vi "ClickOnSquereOperations.vi"(9 "Input DataBase":T1, 10 "Off Board?":bool, 11 "Clicked Position":i32[](array[numeric])) -> (2 "Output DataBase":T1, 3 "Output State":T8)   [LabVIEW 2019]
uses:
  #typedef_DataBase.ctl
  #typedef_SquareType.ctl
  #typedef_Color.ctl
  #typedef_Piece.ctl
  #typedef_PieceType.ctl
  #typedef_SquareLook.ctl
  #typedef_SpecialMoves.ctl
  #typedef_ProgramStates.ctl
panel:
  out "?":u16[][](array[ring])
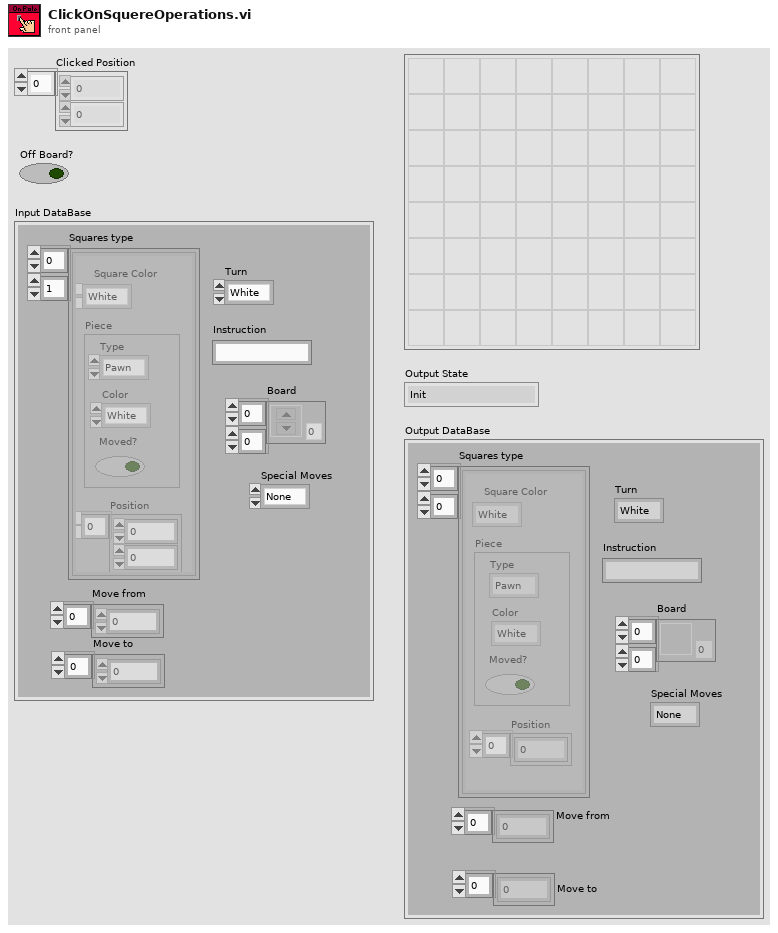
[diagram p1: front panel]
types:
  T1 = typedef "#typedef_DataBase.ctl" = cluster{"Squares type":T2[][], "Turn":T3, "Move from":i32[], "Move to":i32[], "Instruction":string, "Board":T6[][], "Special Moves":T7}
  T2 = typedef "#typedef_SquareType.ctl" = cluster{"Square Color":T3, "Position":i32[], "Piece":T4}
  T3 = typedef "#typedef_Color.ctl" = enum16{"White", "Black"}
  T4 = typedef "#typedef_Piece.ctl" = cluster{"Type":T5, "Color":T3, "Moved?":bool}
  T5 = typedef "#typedef_PieceType.ctl" = enum16{"None", "Pawn", "Knight", "Bishop", "Rook", "Queen", "King"}
  T6 = typedef "#typedef_SquareLook.ctl" = u16
  T7 = typedef "#typedef_SpecialMoves.ctl" = enum16{"None", "Last Square", "Beat in the Passage", "Short Castle", "Long Castle"}
  T8 = typedef "#typedef_ProgramStates.ctl" = enum16{"Init", "Clicking on Piece", "Clicking on Square", "Checking Movement", "Checking King  ", "Checking if Mate", "End"}
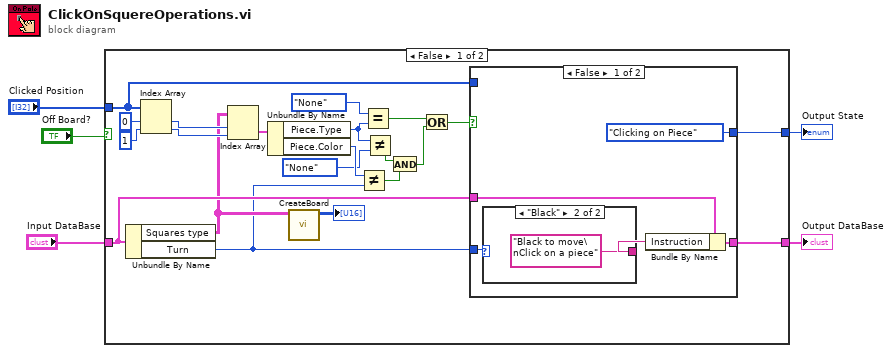
[diagram p0: block diagram]
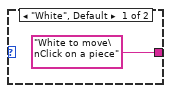
[diagram p2: hidden frame]
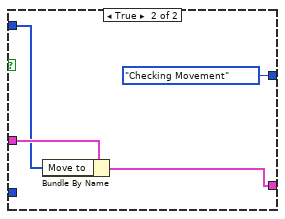
[diagram p3: hidden frame]
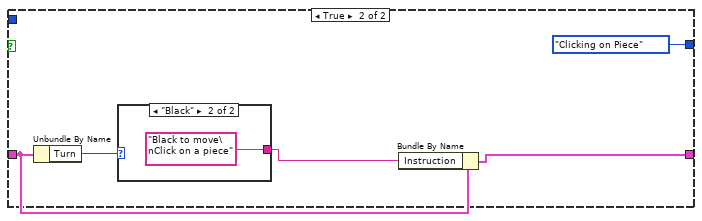
[diagram p4: hidden frame]
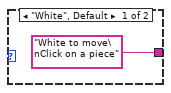
[diagram p5: hidden frame]
diagram:
  n1 = case shown="False" "Off Board?" {
    tunnel: "Input DataBase" -> [w19 w40]
    tunnel: [w18 w38] -> w1
    tunnel: [w20 #typedef_ProgramStates."Clicking on Piece" ("Conditional State")] -> w2
    tunnel: "Clicked Position" -> [w15 _]
    frame False {
      n2 = Unbundle By Name(w19) -> ("Squares type"=w17:T2[][], "Turn"=w12:T3)
      n3 = Index Array(array=w15, index #1=0 ("index"), index #2=1 ("index")) -> (element #1=w24:i32, element #2=w23:i32)
      n4 = Index Array(array=w17, index (row)=w24, index (col)=w23) -> (element=w22:T2)
      n5 = Unbundle By Name(w22) -> ("Piece.Type"=w14:T5, "Piece.Color"=w13:T3)
      n6 = call "CreateBoard.vi"("Squares type"=w17) -> ("Board"=→"?":u16[][])  [unwired: 10 in]
      n7 = Not Equal?(x=w13, y=w12) -> (x != y?=w10:bool)
      n8 = Equal?(x=#typedef_PieceType."None", y=w14) -> (x = y?=w6:bool)
      n9 = Not Equal?(x=w14, y=#typedef_PieceType."None") -> (x != y?=w9:bool)
      n10 = And(x=w9, y=w10) -> (x .and. y?=w7:bool)
      n11 = Or(x=w6, y=w7) -> (x .or. y?=w8:bool)
      n12 = case shown="False" w8 {
        tunnel: [#typedef_ProgramStates."Clicking on Piece" ("Conditional State") #typedef_ProgramStates."Checking Movement" ("Conditional State")] -> w20
        tunnel: w19 -> [w30 w37]
        tunnel: [w29 w36] -> w18
        tunnel: w15 -> [_ w34]
        tunnel: w12 -> [w28 _]
        frame False {
          n13 = case shown="\"Black\"" w28 {
            tunnel: ["White to move\nClick on a piece" "Black to move\nClick on a piece"] -> w27
            frame "White", Default {
            }
            frame "Black" {
            }
          }
          n14 = Bundle By Name(cluster=w30, "Instruction"=w27) -> (w29:T1)
        }
        frame True {
          n15 = Bundle By Name(cluster=w37, "Move to"=w34) -> (w36:T1)
        }
      }
    }
    frame True {
      n16 = Unbundle By Name(w40) -> ("Turn"=w41:T3)
      n17 = case shown="\"Black\"" w41 {
        tunnel: ["White to move\nClick on a piece" "Black to move\nClick on a piece"] -> w39
        frame "White", Default {
        }
        frame "Black" {
        }
      }
      n18 = Bundle By Name(cluster=w40, "Instruction"=w39) -> (w38:T1)
    }
  }
  "Output State" <- w2
  "Output DataBase" <- w1
